vi "DAQmx Create Channel (DI-Digital Input).vi"(0 "task in":refnum<k21>, 5 "lines":tag, 7 "name to assign":string, 9 "line grouping":i32(ring)=1 items=["one channel for each line", "one channel for all lines"], 11 "error in":errorcluster) -> (4 "task out":refnum<k21>, 15 "error out":errorcluster)   [LabVIEW 2020]
doc: "Creates channel(s) to measure digital signals. You can group digital lines into one digital channel or separate them into multiple digital channels. If you specify one or more entire ports in the <B>lines</B> input by using port physical channel names, you cannot separate the ports into multiple channels. To separate ports into multiple channels, use this VI multiple times with a different port each time."
uses:
  nilvaiu.dll
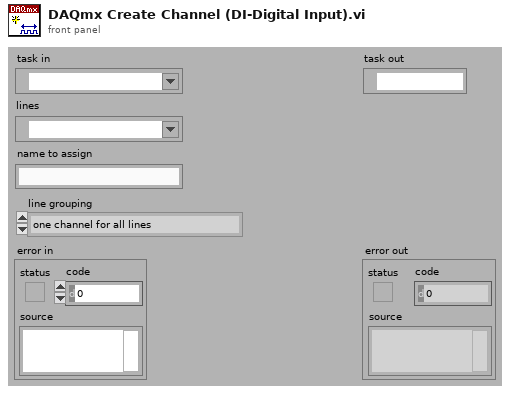
[diagram p1: front panel]
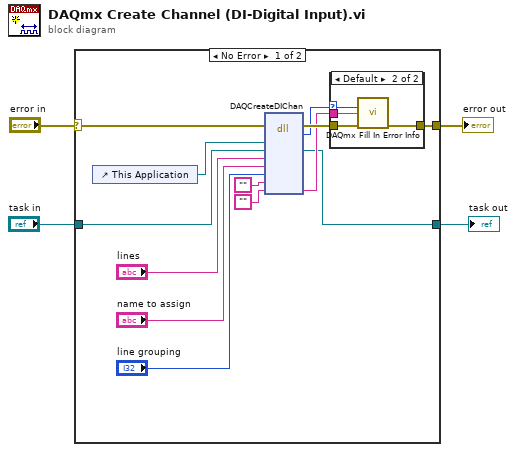
[diagram p0: block diagram]
diagram:
  n1 = case shown="No Error" "error in" {
    selector: "error in" -> [w7 w24]
    tunnel: [w13 w24] -> w4
    tunnel: "task in" -> [w10 w23]
    tunnel: [w9 w23] -> w2
    frame No Error {
      n2 = control-ref of="This Application"() -> (w17:refnum<vi>)
      n3 = dll-call lib="nilvaiu.*" fn="DAQCreateDIChan"(error in=w7, "lvAppRef"=w17, "refObjPtr"=w10, "lines"="lines", "channelNameIn"="name to assign", "lineGrouping"="line grouping", "channelNamesOut"="", "extendedErrorInfo"="") -> (error out=w15:errorcluster, "return type"=w6:i32, "refObjPtr"=w9:refnum<k21>, "extendedErrorInfo"=w14:string)  [unwired: 7 in, 1 out]
      n4 = case shown="Default" w6 {
        selector: w6 -> [_ w19]
        tunnel: w15 -> [w18 w22]
        tunnel: w14 -> [_ w21]
        tunnel: [w18 w20] -> w13
        frame 0 {
        }
        frame Default {
          n5 = call "DAQmx Fill In Error Info.vi"("status code"=w19, "extended error info"=w21, "error in"=w22) -> ("error out"=w20:errorcluster)  [unwired: 1 in, 11 out]
        }
      }
    }
    frame Error {
    }
  }
  "error out" <- w4
  "task out" <- w2
